vi "flatten_var_config.vi"(8 "error in (no error)":errorcluster, 10 "var_config":T1={"hardware"=enum."none", "options"="", "repeats"=1, "loops"=1, "VISA"="", "override_VISA"=FALSE} {"loops" min=1; "repeats" min=1}, 11 "name":string) -> (0 "error out":errorcluster, 1 "values":variant[](array[variant]), 2 "names":string[](array[string]))   [LabVIEW 2017, in "tools.lvlib"]
uses:
  tools.lvlib
  var_config.ctl
  ctrl/var_list.ctl
  <vilib>/Utility/VariantDataType/GetClusterInfo.vi
  <vilib>/Utility/VariantDataType/GetTypeInfo.vi
  <vilib>/UPVI/lvhdf5/attribute.llb/Cluster to Attribute Array.xnode
  <vilib>/Utility/VariantDataType/VariantType.lvlib
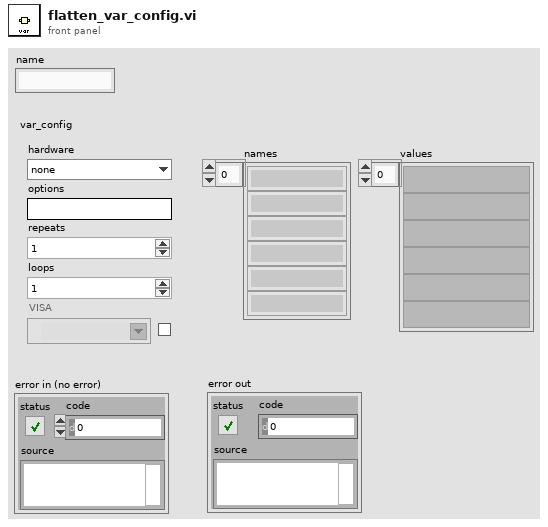
[diagram p1: front panel]
types:
  T1 = typedef "tools.lvlib/var_config.ctl" = cluster{"hardware":T2, "options":string, "repeats":i32, "loops":i32, "VISA":refnum<visa-resource-name>, "override_VISA":bool}
  T2 = typedef "var_list.ctl" = enum16{"none", "AO voltage (V)", "delay (s)", "generic", "microwaves (GHz)", "radiant (nm)", "radiant thg (nm)", "sirah (nm)", "sirah_shg (nm)", "tenma voltage (V)", "wait (s)", "wf_freq (Hz)", "wf_amp (V)", "wf_amp_multi (V)", "wf_offset (V)", "wf_low_level (V)", "wf_high_level (V)", "wf_period (s)", "wf_pulse_width (s)", "wf_sample_rate (Sa/s)", "wf_multi_amp", "wf_multi_freq", "wf_arb_4chan", "WS7 setpoint (nm)"}
  T3 = cluster{"hardware":T2, "options":string, "repeats":i32, "loops":i32}
  T4 = cluster{"hardware":T2, "options":string, "repeats":i32, "loops":i32, "VISA":string}
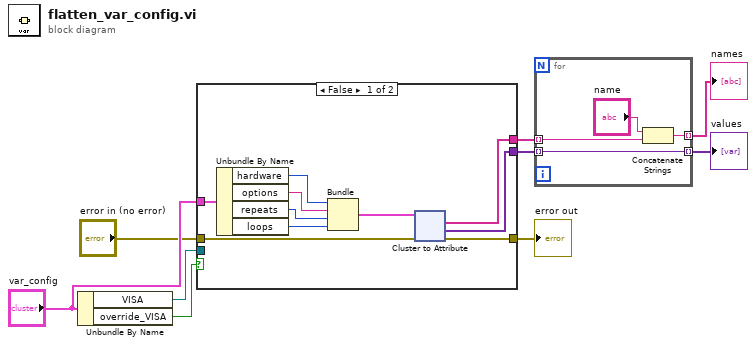
[diagram p0: block diagram]
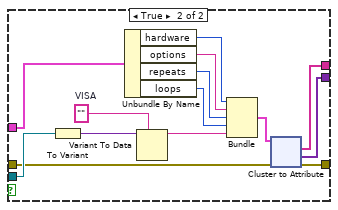
[diagram p2: hidden frame]
diagram:
  n1 = Unbundle By Name("var_config") -> ("VISA"=w4:refnum<visa-resource-name>, "override_VISA"=w9:bool)
  n2 = case shown="False" w9 {
    tunnel: "var_config" -> [w15 w103]
    tunnel: [w13 w112] -> w8
    tunnel: [w12 w111] -> w7
    tunnel: w4 -> [_ w110]
    tunnel: "error in (no error)" -> [w10 w102]
    tunnel: [w11 w101] -> w1
    frame False {
      n3 = Unbundle By Name(w15) -> ("hardware"=w16:T2, "options"=w17:string, "repeats"=w18:i32, "loops"=w19:i32)
      n4 = Bundle("hardware"=w16, "options"=w17, "repeats"=w18, "loops"=w19) -> (w14:T3)  [unwired: 1 in]
      n5 = xnode "Cluster to Attribute"("error in (no error)"=w10, "Cluster"=w14) -> ("Names out"=w13:string[], "Values out"=w12:variant[], "error out"=w11:errorcluster)  [unwired: 4 in]
    }
    frame True {
      w114 = ""  # VISA
      n6 = To Variant(anything=w110) -> (Variant=w113:variant)
      n7 = Unbundle By Name(w103) -> ("hardware"=w106:T2, "options"=w107:string, "repeats"=w108:i32, "loops"=w109:i32)
      n8 = Variant To Data(type=w114, Variant=w113) -> (data=w105:string)  [unwired: 1 in, 1 out]
      n9 = Bundle("hardware"=w106, "options"=w107, "repeats"=w108, "loops"=w109, "VISA"=w105) -> (w104:T4)  [unwired: 1 in]
      n10 = xnode "Cluster to Attribute"("error in (no error)"=w102, "Cluster"=w104) -> ("Names out"=w112:string[], "Values out"=w111:variant[], "error out"=w101:errorcluster)  [unwired: 4 in]
    }
  }
  "error out" <- w1
  n11 = for {
    tunnel: w8 -> [w201] mode=indexing
    tunnel: [w200] -> w6 mode=indexing
    tunnel: w7 -> [w199] mode=indexing
    tunnel: [w199] -> w5 mode=indexing
    n12 = Concatenate Strings("name", w201) -> (w200:string)
  }
  "values" <- w5
  "names" <- w6
